vi "sub_main_gmap.vi"(8 "error in":errorcluster) -> (0 "error out":errorcluster)   [LabVIEW 2019]
uses:
  Gmap/gmap_fgv-cmd.ctl
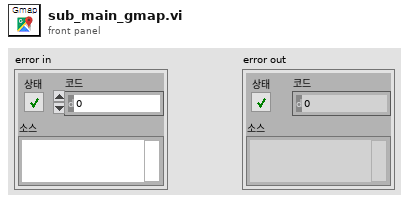
[diagram p1: front panel]
types:
  T1 = typedef "gmap_fgv-cmd.ctl" = enum16{"marker type change", "save_image", "coll of points", "zoom n center markers", "add overlay reference", "read", "zoom", "set position by keyword", "set map provider", "map provider update", "create", "add marker", "clear marker", "close"}
  T2 = cluster{"AGV":u16, "AGV Estop":u16, "Obstacle":u16, "Heading":u16, "Waypt":u16, "GNSS":u16, "VLP16":u16, "Cam":u16, "RPLidar":u16, "Joystick":u16, "IMU":u16}
  T3 = cluster{"zoom":dbl, "dt clear":u32, "dt add ":u32, "PinDropMrkr":enum16{"none", "arrow", "blue", "blue_small", "blue_dot", "blue_pushpin", "brown_small", "gray_small", "green", "green_small", "green_dot", "green_pushpin", "green_big_go", "yellow", "yellow_small", "yellow_dot", "yellow_big_pause", "yellow_pushpin", "lightblue", "lightblue_dot", "lightblue_pushpin", "orange", "orange_small", "orange_dot", "pink", "pink_dot", "pink_pushpin", "purple", "purple_small", "purple_dot", "purple_pushpin", "red", "red_small", "red_dot", "red_pushpin", "red_big_stop", "black_small", "white_small"}, "zoom n center":bool}
  T4 = enum16{"none", "arrow", "blue", "blue_small", "blue_dot", "blue_pushpin", "brown_small", "gray_small", "green", "green_small", "green_dot", "green_pushpin", "green_big_go", "yellow", "yellow_small", "yellow_dot", "yellow_big_pause", "yellow_pushpin", "lightblue", "lightblue_dot", "lightblue_pushpin", "orange", "orange_small", "orange_dot", "pink", "pink_dot", "pink_pushpin", "purple", "purple_small", "purple_dot", "purple_pushpin", "red", "red_small", "red_dot", "red_pushpin", "red_big_stop", "black_small", "white_small"}
  T5 = cluster{"latlong out":dbl[], "PinDropMrkr":enum16{"none", "arrow", "blue", "blue_small", "blue_dot", "blue_pushpin", "brown_small", "gray_small", "green", "green_small", "green_dot", "green_pushpin", "green_big_go", "yellow", "yellow_small", "yellow_dot", "yellow_big_pause", "yellow_pushpin", "lightblue", "lightblue_dot", "lightblue_pushpin", "orange", "orange_small", "orange_dot", "pink", "pink_dot", "pink_pushpin", "purple", "purple_small", "purple_dot", "purple_pushpin", "red", "red_small", "red_dot", "red_pushpin", "red_big_stop", "black_small", "white_small"}}
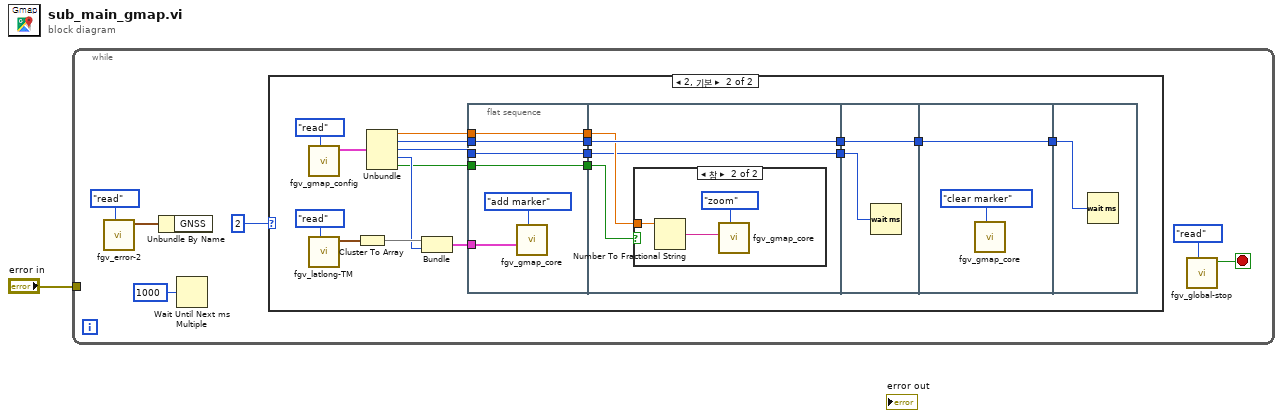
[diagram p0: block diagram]
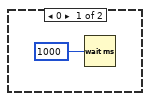
[diagram p2: hidden frame]
diagram:
  n1 = while {
    tunnel: "error in" -> [_]
    stop <- w3 stop-if-true
    n2 = call "fgv_error-2.vi"("cmd"=enum16{"init", "read", "write"}."read") -> ("Error cluster out"=w6:T2)  [unwired: 9 in, 1 out]
    n3 = Unbundle By Name(w6) -> ()  [unwired: 1 out]
    n4 = Wait Until Next ms Multiple(millisecond multiple=u32 1000 ("ms 배수")) -> ()  [unwired: 1 out]
    n5 = case shown="2, 기본" u16 2 ("GNSS") {
      frame 0 {
        n6 = Wait (ms)(milliseconds to wait=u32 1000 ("대기 시간 (ms)")) -> ()  [unwired: 1 out]
      }
      frame 2, Default {
        n7 = call "fgv_gmap_config.vi"("cmd"=enum16{"read", "write"}."read") -> ("gmap cfg out"=w23:T3)  [unwired: 9 in, 1 out]
        n8 = call "fgv_latlong-TM.vi"("cmd"=enum16{"write", "read"}."read") -> ("latlong out"=w9:cluster{"lat":dbl, "long":dbl})  [unwired: 9 in, 1 out]
        n9 = Cluster To Array(cluster=w9) -> (array=w27:dbl[])
        n10 = Unbundle(w23) -> ("zoom"=w19:dbl, "dt clear"=w20:u32, "dt add"=w12:u32, "PinDropMrkr"=w17:T4, "zoom n center"=w10:bool)
        n11 = Bundle("latlong out"=w27, "PinDropMrkr"=w17) -> (w25:T5)  [unwired: 1 in]
        n12 = flat-sequence {
          tunnel: [w31] -> w21
          tunnel: [w30] -> w18
          tunnel: w19 -> [w30]
          tunnel: w20 -> [w31]
          tunnel: w25 -> [w32]
          tunnel: [w29] -> w13
          tunnel: w12 -> [w29]
          tunnel: [w28] -> w11
          tunnel: w10 -> [w28]
          tunnel: [w37] -> w22
          tunnel: w21 -> [w37]
          tunnel: w18 -> [w36]
          tunnel: [w35] -> w14
          tunnel: w13 -> [w35]
          tunnel: w11 -> [w34]
          tunnel: w22 -> [w42]
          tunnel: [w42] -> w15
          tunnel: w14 -> [w41]
          tunnel: [w43] -> w16
          tunnel: w15 -> [w43]
          tunnel: w16 -> [w45]
          frame #0 {
            n13 = call "fgv_gmap_core.vi"("cmd"=gmap_fgv-cmd."add marker", "marker_info"=w32) -> ()  [unwired: 6 in, 4 out]
          }
          frame #1 {
            n14 = case shown="참" w34 {
              tunnel: w36 -> [_ w38]
              frame False {
              }
              frame True {
                n15 = Number To Fractional String(number=w38) -> (F-format string=w39:string)  [unwired: 3 in]
                n16 = call "fgv_gmap_core.vi"(7:"cmd"=gmap_fgv-cmd."zoom" ("cmd"), 10:"cmd"=w39) -> ()  [unwired: 6 in, 4 out]
              }
            }
          }
          frame #2 {
            n17 = Wait (ms)(milliseconds to wait=w41) -> ()  [unwired: 1 out]
          }
          frame #3 {
            n18 = call "fgv_gmap_core.vi"("cmd"=gmap_fgv-cmd."clear marker") -> ()  [unwired: 7 in, 4 out]
          }
          frame #4 {
            n19 = Wait (ms)(milliseconds to wait=w45) -> ()  [unwired: 1 out]
          }
        }
      }
    }
    n20 = call "fgv_global-stop.vi"("cmd"=enum16{"init", "stop", "read"}."read") -> ("val_out"=w3:bool)  [unwired: 10 in]
  }
